vi "ThingWorxInit.vi"(9 "Properties":string[](array[string]), 11 "Input Array":string[](array[string])) -> (0 "Properties Out":string[](array[string]), 1 "Service Name":string, 2 "appKey":string, 3 "url beginning":string)   [LabVIEW 2015]
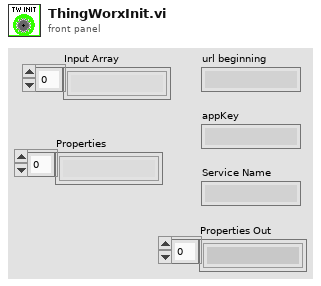
[diagram p1: front panel]
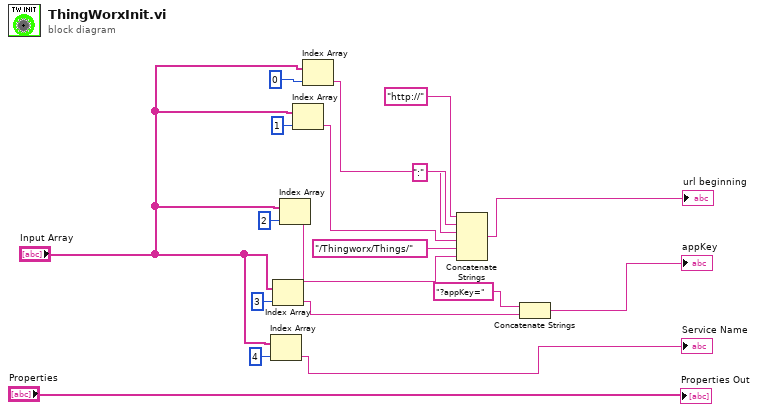
[diagram p0: block diagram]
diagram:
  n1 = Index Array(array="Input Array", index=4) -> (element=→"Service Name":string)
  n2 = Index Array(array="Input Array", index=3) -> (element=w15:string)
  n3 = Index Array(array="Input Array", index=2) -> (element=w13:string)
  n4 = Index Array(array="Input Array", index=1) -> (element=w11:string)
  n5 = Index Array(array="Input Array", index=0) -> (element=w10:string)
  n6 = Concatenate Strings("http://" ("url"), w10, ":" ("url"), w11, "/Thingworx/Things/" ("url"), w13) -> (→"url beginning":string)
  n7 = Concatenate Strings("?appKey=" ("url"), w15) -> (→"appKey":string)
  "Properties Out" <- "Properties"
